vi "boc_measure_all_channels.vi"(7 "Function":T11, 8 "error in (no error)":errorcluster, 9 "current_channel":i32, 10 "paramUnicorn in":T1, 11 "input cluster":T8) -> (0 "error out":errorcluster, 1 "boc_values":sgl[](array[numeric]), 2 "paramUnicorn out":T1, 3 "output cluster":T8, 5 "results":dbl[](array[numeric]))   [LabVIEW 2017]
uses:
  <instrlib>/PICOTEST M352XA/Public/Controls/Function.ctl
  ui.ctl
  classes/dc_power_supply/DC_power_supply.lvclass
  classes/report/Report.lvclass
  ui_buttons.ctl
  types/boc_type.ctl
  Unicorn Labview Library/Control/unicorn_Param.ctl
  Unicorn Labview Library/Control/unicorn_conn.ctl
  Unicorn Labview Library/Control/unicorn_JSON.ctl
  Unicorn Labview Library/Control/unicorn_ParamInt.ctl
  Unicorn Labview Library/Control/unicorn_Telemetry.ctl
  Unicorn Labview Library/Control/unicorn_Table.ctl
  Unicorn Labview Library/Control/unicorn_ParamFloat.ctl
  Unicorn Labview Library/Unicorn Library.lvlib
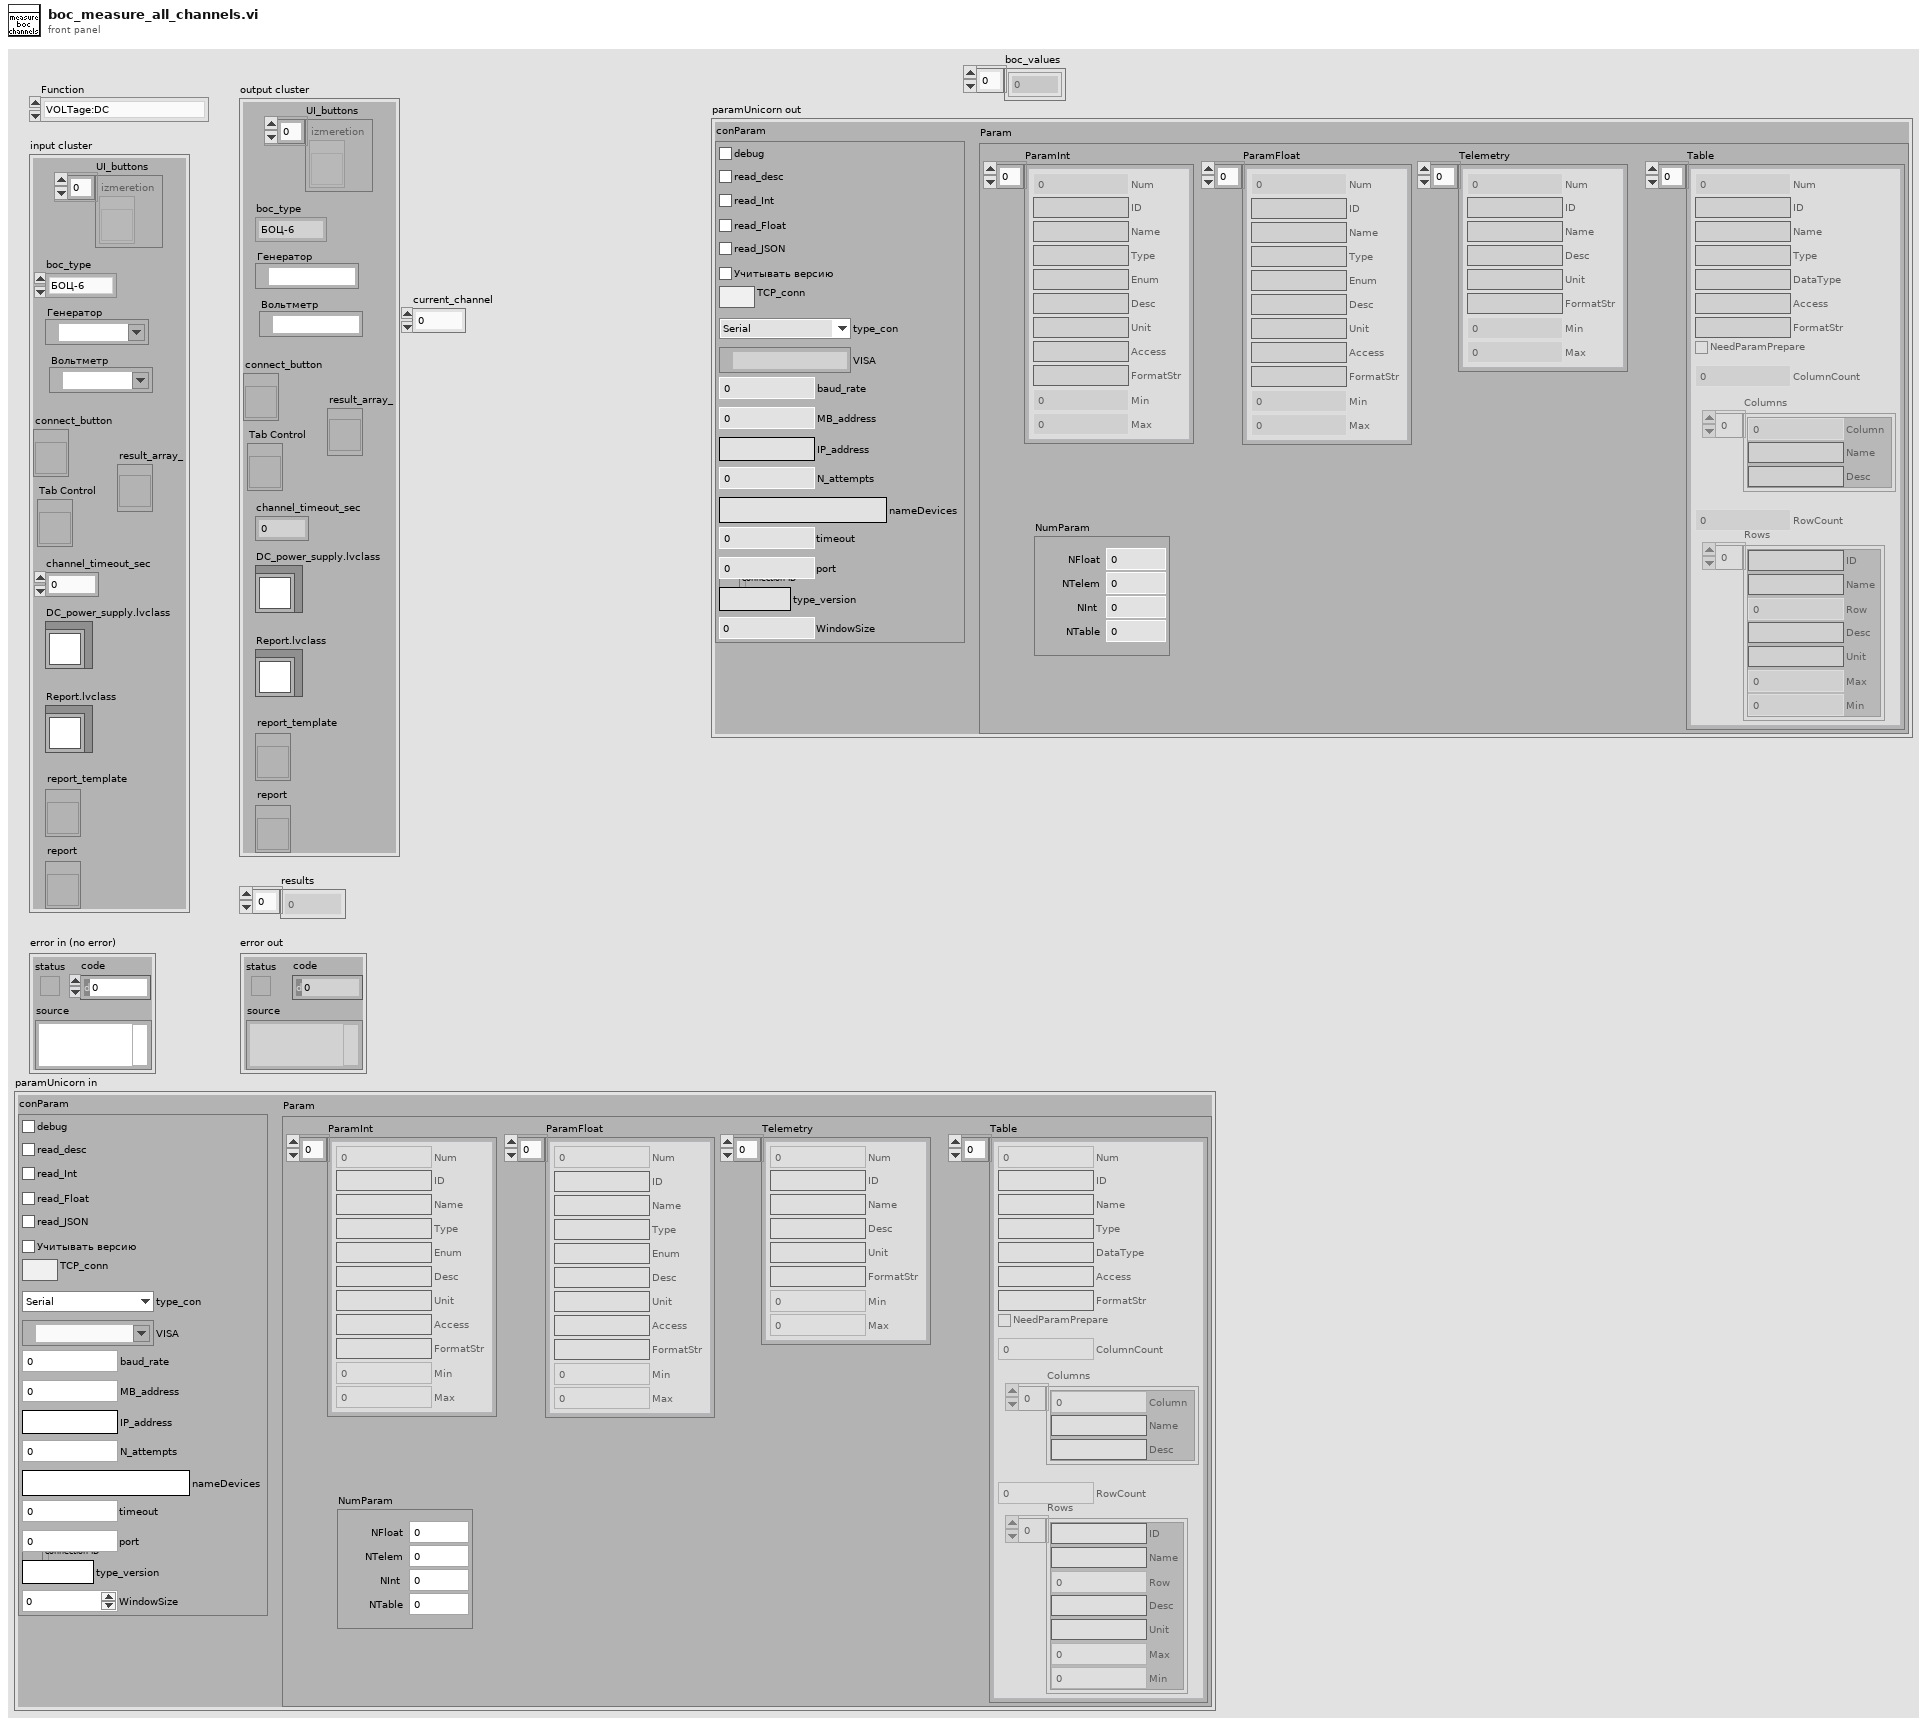
[diagram p1: front panel]
types:
  T1 = typedef "Unicorn Library.lvlib/unicorn_Param.ctl" = cluster{"conParam":T2, "Param":T3}
  T2 = typedef "Unicorn Library.lvlib/unicorn_conn.ctl" = cluster{"ReadIntParam":bool, "ReadDescrParam":bool, "ReadFloatParam":bool, "debug":bool, "ReadJSON":bool, "IP_address":string, "N_attempts":i32, "type_con":enum16{"Serial", "TCP"}, "MB_address":i32, "VISA":refnum<visa-resource-name>, "connection ID":refnum<k5>, "nameDevices":string, "timeout":i32, "port":u16, "type_version":string, "baud_rate":u32, "VersionControl":bool, "TCP_conn":bool, "WindowSize":i32}
  T3 = typedef "Unicorn Library.lvlib/unicorn_JSON.ctl" = cluster{"NumParam":cluster{"NTelem":i32, "NInt":i32, "NFloat":i32, "NTable":i32}, "ParamInt":T4, "Telemetry":T5, "Table":T6, "ParamFloat":T7}
  T4 = typedef "Unicorn Library.lvlib/unicorn_ParamInt.ctl" = cluster{"ID":string, "Num":i32, "Name":string, "Type":string, "Enum":string, "Desc":string, "Unit":string, "Access":string, "FormatStr":string, "Min":i32, "Max":i32}[]
  T5 = typedef "Unicorn Library.lvlib/unicorn_Telemetry.ctl" = cluster{"ID":string, "Num":i32, "Name":string, "Desc":string, "Unit":string, "FormatStr":string, "Min":i32, "Max":i32}[]
  T6 = typedef "Unicorn Library.lvlib/unicorn_Table.ctl" = cluster{"Num":i32, "Access":string, "ColumnCount":i32, "NeedParamPrepare":bool, "Columns":cluster{"Column":i32, "Desc":string, "Name":string}[], "DataType":string, "FormatStr":string, "ID":string, "Name":string, "RowCount":i32, "Rows":cluster{"Desc":string, "ID":string, "Max":i32, "Min":i32, "Name":string, "Row":i32, "Unit":string}[], "Type":string}[]
  T7 = typedef "Unicorn Library.lvlib/unicorn_ParamFloat.ctl" = cluster{"ID":string, "Num":i32, "Name":string, "Type":string, "Enum":string, "Desc":string, "Unit":string, "Access":string, "FormatStr":string, "Min":i32, "Max":i32}[]
  T8 = typedef "ui.ctl" = cluster{"UI_buttons":T9, "Tab Control":refnum<vi>, "connect_button":refnum<vi>, "generator":refnum<visa-resource-name>, "voltmetr":refnum<visa-resource-name>, "channel_timeout_sec":dbl, "boc_type":T10, "result_array_":refnum<vi>, "DC_power_supply.lvclass":refnum<class "DC_power_supply.lvclass">, "Report.lvclass":refnum<class "Report.lvclass">, "report_template":refnum<vi>, "report":refnum<vi>}
  T9 = typedef "ui_buttons.ctl" = refnum<vi>[]
  T10 = typedef "boc_type.ctl" = enum16{"БОЦ-6", "БОЦ-12"}
  T11 = typedef "Function.ctl" = enum16{"VOLTage:DC", "VOLTage:DC:RATio", "VOLTage:AC", "CURRent:DC", "CURRent:AC", "RESistance", "FRESistance", "FREQuency", "PERiod", "FREQuency:CURRent", "PERiod:CURRent", "CAPacitance", "CONTinuity", "DIODe", "TCOuple", "TEMPerature"}
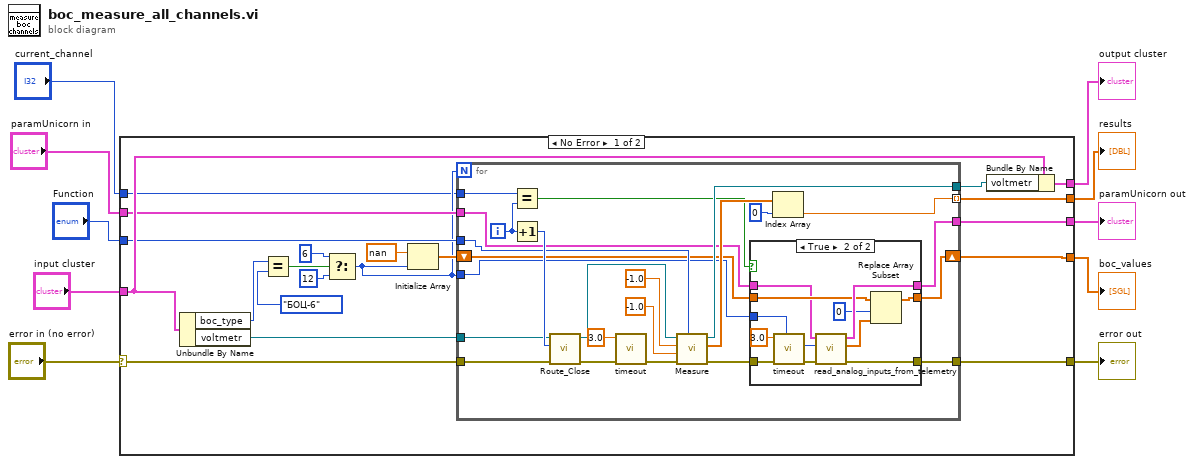
[diagram p0: block diagram]
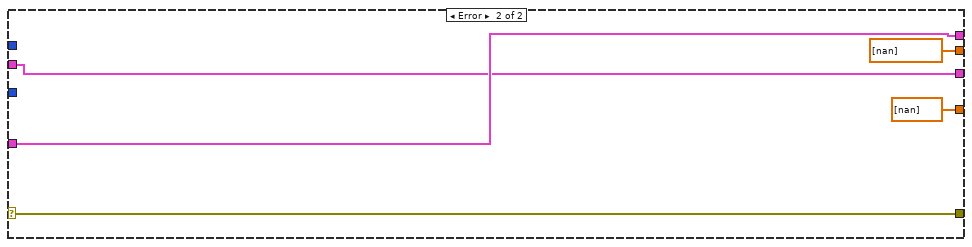
[diagram p3: hidden frame]
diagram:
  n1 = case shown="No Error" "error in (no error)" {
    selector: "error in (no error)" -> [w21 w71]
    tunnel: "input cluster" -> [w30 w73]
    tunnel: [w29 w73] -> w9
    tunnel: [w28 dbl[] [nan]] -> w8
    tunnel: "Function" -> [w26 _]
    tunnel: "paramUnicorn in" -> [w13 w69]
    tunnel: [w18 w71] -> w4
    tunnel: [w17 sgl[] [nan] ("values")] -> w3
    tunnel: [w16 w69] -> w2
    tunnel: "current_channel" -> [w11 _]
    frame No Error {
      n2 = Unbundle By Name(w30) -> ("boc_type"=w19:T10, "voltmetr"=w25:refnum<visa-resource-name>)
      n3 = Equal?(x=w19, y=enum16{"БОЦ-6", "БОЦ-12"}."БОЦ-6") -> (x = y?=w22:bool)
      n4 = Select(t=u8 6, s=w22, f=u8 12) -> (s? t:f=w12:u8)
      n5 = Initialize Array(nan ("element"), w12) -> (w14:dbl[])
      n6 = for {
        N: w12 -> [_]
        tunnel: w21 -> [w53]
        tunnel: w25 -> [w42]
        tunnel: w26 -> [w47]
        tunnel: [w46] -> w27
        tunnel: [w43] -> w28 mode=indexing
        tunnel: w12 -> [w39]
        tunnel: [w38] -> w18
        tunnel: [w37] -> w16
        shift-right: [w33] -> w17
        shift-left: w14 -> [w34]
        tunnel: w13 -> [w32]
        tunnel: w11 -> [w31]
        i -> [w36]
        n7 = Equal?(x=w31, y=w36) -> (x = y?=w35:bool)
        n8 = Increment(x=w36) -> (x+1=w54:i32)
        n9 = call <instrlib>:"Route_Close.vi"("error in (no error)"=w53, "channel"=w54, "VISA resource name"=w42) -> ("error out"=w52:errorcluster, "VISA resource name out"=w41:refnum<visa-resource-name>)  [unwired: 6 in, 1 out]
        n10 = call "timeout.vi"("error in (no error)"=w52, "seconds to wait"=3.0) -> ("error IO"=w50:errorcluster)  [unwired: 9 in]
        n11 = call <instrlib>:"Measure.vi"("Function"=w47, "error in (no error)"=w50, "Resolution"=-1.0, "Range"=-1.0, "VISA resource name"=w41) -> ("error out"=w40:errorcluster, "Measurements"=w45:dbl[], "VISA resource name out"=w46:refnum<visa-resource-name>)  [unwired: 4 in]
        n12 = case shown="True" w35 {
          tunnel: w40 -> [w57 w60]
          tunnel: w39 -> [_ w68]
          tunnel: [w57 w67] -> w38
          tunnel: [w55 w66] -> w37
          tunnel: w34 -> [w56 w65]
          tunnel: [w56 w62] -> w33
          tunnel: w32 -> [w55 w61]
          frame False {
          }
          frame True {
            n13 = call "timeout.vi"("error in (no error)"=w60, "seconds to wait"=3.0) -> ("error IO"=w59:errorcluster)  [unwired: 9 in]
            n14 = call "read_analog_inputs_from_telemetry.vi"("error_in"=w59, "channel_count"=w68, "paramUnicorn in"=w61) -> ("error_out"=w67:errorcluster, "values"=w64:sgl[], "paramUnicorn out"=w66:T1)  [unwired: 6 in]
            n15 = Replace Array Subset(array=w65, new element=w64, index=0) -> (w62:dbl[])
          }
        }
        n16 = Index Array(array=w45, index=0) -> (element=w43:dbl)
      }
      n17 = Bundle By Name(cluster=w30, "voltmetr"=w27) -> (w29:T8)
    }
    frame Error {
    }
  }
  "error out" <- w4
  "results" <- w8
  "output cluster" <- w9
  "boc_values" <- w3
  "paramUnicorn out" <- w2
